vi "Test Snake Cannot Reverse Horizontally.vi"(8 "error in (no error)":errorcluster, 11 "Test Case In":refnum<class "Snake Test.lvclass">) -> (0 "error out":errorcluster, 3 "Test Case Out":refnum<class "Snake Test.lvclass">)   [LabVIEW 2020, in "Snake Test.lvclass"]
uses:
  Snake Test.lvclass
  Snake Test.lvclass/Snake Test.ctl
  source/Snake/Snake.lvclass
  source/Particle/Position.ctl
  source/Particle.lvclass
  <vilib>/Astemes/LUnit/Test Case.lvclass
  source/Snake/Direction.ctl
  C:/Program Files (x86)/National Instruments/LabVIEW 2020/vi.lib/Astemes/LUnit/Test Case.lvclass
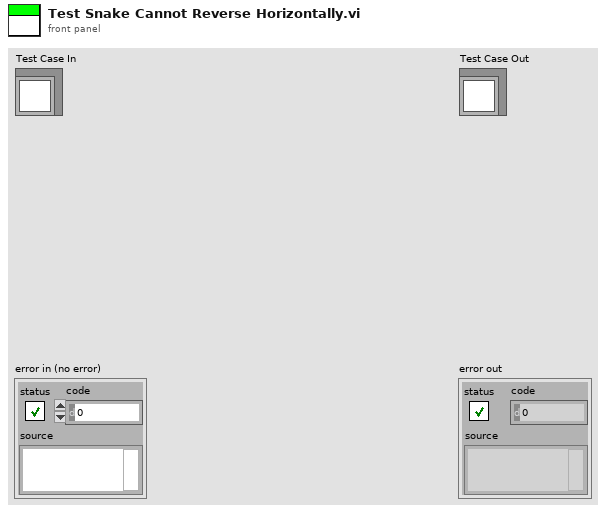
[diagram p1: front panel]
types:
  T1 = typedef "Direction.ctl" = enum16{"X", "-X", "Y", "-Y"}
  T2 = typedef "Particle.lvclass/Position.ctl" = cluster{"X":i32, "Y":i32}
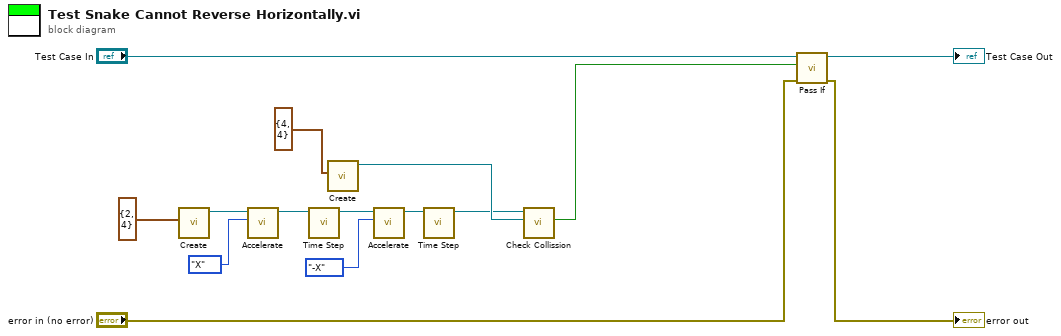
[diagram p0: block diagram]
diagram:
  n1 = call "Create.vi"("Position"=T2 {"X"=2, "Y"=4}) -> ("Snake out"=w11:refnum<class "Snake.lvclass">)  [unwired: 10 in]
  n2 = call "Accelerate.vi"("Direction"=enum16{"X", "-X", "Y", "-Y"}."X", "Snake in"=w11) -> ("Snake out"=w5:refnum<class "Snake.lvclass">)  [unwired: 9 in]
  n3 = call "Time Step.vi"("Snake in"=w5) -> ("Snake out"=w4:refnum<class "Snake.lvclass">)  [unwired: 10 in]
  n4 = call "Create.vi"("Position"=T2 {"X"=4, "Y"=4}) -> ("Particle out"=w9:refnum<class "Particle.lvclass">)  [unwired: 10 in]
  n5 = call "Accelerate.vi"("Direction"=Direction."-X", "Snake in"=w4) -> ("Snake out"=w3:refnum<class "Snake.lvclass">)  [unwired: 9 in]
  n6 = call "Time Step.vi"("Snake in"=w3) -> ("Snake out"=w2:refnum<class "Snake.lvclass">)  [unwired: 10 in]
  n7 = call "Check Collission.vi"("Particle"=w9, "Snake in"=w2) -> ("Collided?"=w8:bool)  [unwired: 8 in, 1 out]
  n8 = call <vilib>:"Pass If.vi"("error in (no error)"="error in (no error)", "Pass?"=w8, "LUnit Test Case In"="Test Case In") -> ("error out"=→"error out":errorcluster, "LUnit Test Case Out"=→"Test Case Out":refnum<class "Snake Test.lvclass">)  [unwired: 7 in]
